vi "gui.vi"(8 "dx":dbl=0.005 format="%#_13g", 9 "f(x)":string[](array[string])=["-sin(x*2*pi(1)) ", "-abs(sin(x*2*pi(1)))", "sin(x*2*pi(1))", "abs(sin(x*2*pi(1)))"], 10 "N":i32=201) -> (2 "y_vals":dbl[][](array[numeric])=[[2.4492935982947064e-16, -0.03141075907812698, -0.06279051952931278, -0.09410831331851353, -0.12533323356430418, -0.15643446504022973, -0.1873813145857242, -0.21814324139654195, -0.24868988716485488, -0.27899110603922833, -0.3090169943749472, -0.338737920245291, -0.3681245526846782, -0.3971478906347799, -0.42577929156507255, -0.4539904997395466, -0.48175367410171566, -0.5090414157503708, -0.5358267949789967, -0.5620833778521305, -0.5877852522924736, -0.6129070536529762, -0.6374239897486899, -0.6613118653236519, -0.6845471059286893, -0.7071067811865474, -0.7289686274214106, -0.7501110696304591, -0.7705132427757893, -0.7901550123756903, -0.8090169943749468, -0.8270805742745616, -0.8443279255020147, -0.8607420270039436, -0.8763066800438631, -0.8910065241883677, -0.9048270524660194, -0.9177546256839813, -0.9297764858882511, -0.9408807689542255, -0.9510565162951535, -0.9602936856769432, -0.968583161128631, -0.9759167619387474, -0.9822872507286886, -0.9876883405951378, -0.9921147013144778, -0.99556196460308, -0.9980267284282716, -0.9995065603657316, -1.0, -0.9995065603657316, -0.9980267284282716, -0.99556196460308, -0.9921147013144779, -0.9876883405951379, -0.9822872507286886, -0.9759167619387473, -0.9685831611286311, -0.9602936856769431, -0.9510565162951536, -0.9408807689542257, -0.9297764858882517, -0.9177546256839815, -0.9048270524660192, -0.8910065241883685, -0.8763066800438634, -0.8607420270039435, -0.8443279255020151, -0.8270805742745619, -0.8090169943749477, -0.7901550123756906, -0.7705132427757897, -0.7501110696304601, -0.728968627421411, -0.7071067811865483, -0.6845471059286897, -0.6613118653236517, -0.6374239897486897, -0.6129070536529766, -0.5877852522924734, -0.562083377852131, -0.5358267949789957, -0.5090414157503721, -0.4817536741017162, -0.4539904997395463, -0.42577929156507394, -0.39714789063478045, -0.368124552684678, -0.33873792024529153, -0.3090169943749478, -0.2789911060392298, -0.2486898871648555, -0.21814324139654168, -0.18738131458572568, -0.15643446504023034, -0.1253332335643039, -0.09410831331851592, -0.06279051952931339, -0.03141075907812848, -3.6739403974420594e-16, 0.03141075907812775, 0.06279051952931265, 0.09410831331851519, 0.12533323356430318, 0.15643446504022962, 0.18738131458572496, 0.2181432413965427, 0.24868988716485477, 0.27899110603922905, 0.30901699437494706, 0.33873792024529253, 0.36812455268467725, 0.3971478906347798, 0.42577929156507327, 0.45399049973954725, 0.48175367410171555, 0.5090414157503714, 0.5358267949789951, 0.5620833778521305, 0.5877852522924728, 0.612907053652976, 0.6374239897486891, 0.6613118653236512, 0.6845471059286892, 0.7071067811865479, 0.7289686274214106, 0.7501110696304596, 0.7705132427757893, 0.7901550123756902, 0.8090169943749472, 0.8270805742745615, 0.8443279255020156, 0.8607420270039432, 0.876306680043863, 0.8910065241883681, 0.9048270524660197, 0.9177546256839811, 0.9297764858882513, 0.9408807689542253, 0.951056516295154, 0.960293685676943, 0.968583161128631, 0.9759167619387472, 0.9822872507286885, 0.9876883405951378, 0.9921147013144779, 0.9955619646030799, 0.9980267284282716, 0.9995065603657316, 1.0, 0.9995065603657316, 0.9980267284282716, 0.9955619646030799, 0.992114701314478, 0.9876883405951379, 0.9822872507286886, 0.9759167619387473, 0.9685831611286312, 0.9602936856769432, 0.9510565162951538, 0.9408807689542251, 0.9297764858882517, 0.9177546256839816, 0.9048270524660192, 0.8910065241883677, 0.8763066800438635, 0.8607420270039436, 0.8443279255020161, 0.8270805742745619, 0.8090169943749477, 0.7901550123756907, 0.7705132427757897, 0.7501110696304601, 0.7289686274214111, 0.7071067811865485, 0.6845471059286898, 0.6613118653236518, 0.6374239897486897, 0.6129070536529767, 0.5877852522924735, 0.5620833778521311, 0.5358267949789958, 0.5090414157503722, 0.4817536741017163, 0.4539904997395464, 0.42577929156507244, 0.39714789063478056, 0.3681245526846781, 0.33873792024529165, 0.3090169943749462, 0.2789911060392299, 0.2486898871648556, 0.21814324139654354, 0.1873813145857258, 0.15643446504023048, 0.125333233564304, 0.09410831331851605, 0.06279051952931351, 0.031410759078128604, 4.898587196589413e-16], [-2.4492935982947064e-16, -0.03141075907812698, -0.06279051952931278, -0.09410831331851353, -0.12533323356430418, -0.15643446504022973, -0.1873813145857242, -0.21814324139654195, -0.24868988716485488, -0.27899110603922833, -0.3090169943749472, -0.338737920245291, -0.3681245526846782, -0.3971478906347799, -0.42577929156507255, -0.4539904997395466, -0.48175367410171566, -0.5090414157503708, -0.5358267949789967, -0.5620833778521305, -0.5877852522924736, -0.6129070536529762, -0.6374239897486899, -0.6613118653236519, -0.6845471059286893, -0.7071067811865474, -0.7289686274214106, -0.7501110696304591, -0.7705132427757893, -0.7901550123756903, -0.8090169943749468, -0.8270805742745616, -0.8443279255020147, -0.8607420270039436, -0.8763066800438631, -0.8910065241883677, -0.9048270524660194, -0.9177546256839813, -0.9297764858882511, -0.9408807689542255, -0.9510565162951535, -0.9602936856769432, -0.968583161128631, -0.9759167619387474, -0.9822872507286886, -0.9876883405951378, -0.9921147013144778, -0.99556196460308, -0.9980267284282716, -0.9995065603657316, -1.0, -0.9995065603657316, -0.9980267284282716, -0.99556196460308, -0.9921147013144779, -0.9876883405951379, -0.9822872507286886, -0.9759167619387473, -0.9685831611286311, -0.9602936856769431, -0.9510565162951536, -0.9408807689542257, -0.9297764858882517, -0.9177546256839815, -0.9048270524660192, -0.8910065241883685, -0.8763066800438634, -0.8607420270039435, -0.8443279255020151, -0.8270805742745619, -0.8090169943749477, -0.7901550123756906, -0.7705132427757897, -0.7501110696304601, -0.728968627421411, -0.7071067811865483, -0.6845471059286897, -0.6613118653236517, -0.6374239897486897, -0.6129070536529766, -0.5877852522924734, -0.562083377852131, -0.5358267949789957, -0.5090414157503721, -0.4817536741017162, -0.4539904997395463, -0.42577929156507394, -0.39714789063478045, -0.368124552684678, -0.33873792024529153, -0.3090169943749478, -0.2789911060392298, -0.2486898871648555, -0.21814324139654168, -0.18738131458572568, -0.15643446504023034, -0.1253332335643039, -0.09410831331851592, -0.06279051952931339, -0.03141075907812848, -3.6739403974420594e-16, -0.03141075907812775, -0.06279051952931265, -0.09410831331851519, -0.12533323356430318, -0.15643446504022962, -0.18738131458572496, -0.2181432413965427, -0.24868988716485477, -0.27899110603922905, -0.30901699437494706, -0.33873792024529253, -0.36812455268467725, -0.3971478906347798, -0.42577929156507327, -0.45399049973954725, -0.48175367410171555, -0.5090414157503714, -0.5358267949789951, -0.5620833778521305, -0.5877852522924728, -0.612907053652976, -0.6374239897486891, -0.6613118653236512, -0.6845471059286892, -0.7071067811865479, -0.7289686274214106, -0.7501110696304596, -0.7705132427757893, -0.7901550123756902, -0.8090169943749472, -0.8270805742745615, -0.8443279255020156, -0.8607420270039432, -0.876306680043863, -0.8910065241883681, -0.9048270524660197, -0.9177546256839811, -0.9297764858882513, -0.9408807689542253, -0.951056516295154, -0.960293685676943, -0.968583161128631, -0.9759167619387472, -0.9822872507286885, -0.9876883405951378, -0.9921147013144779, -0.9955619646030799, -0.9980267284282716, -0.9995065603657316, -1.0, -0.9995065603657316, -0.9980267284282716, -0.9955619646030799, -0.992114701314478, -0.9876883405951379, -0.9822872507286886, -0.9759167619387473, -0.9685831611286312, -0.9602936856769432, -0.9510565162951538, -0.9408807689542251, -0.9297764858882517, -0.9177546256839816, -0.9048270524660192, -0.8910065241883677, -0.8763066800438635, -0.8607420270039436, -0.8443279255020161, -0.8270805742745619, -0.8090169943749477, -0.7901550123756907, -0.7705132427757897, -0.7501110696304601, -0.7289686274214111, -0.7071067811865485, -0.6845471059286898, -0.6613118653236518, -0.6374239897486897, -0.6129070536529767, -0.5877852522924735, -0.5620833778521311, -0.5358267949789958, -0.5090414157503722, -0.4817536741017163, -0.4539904997395464, -0.42577929156507244, -0.39714789063478056, -0.3681245526846781, -0.33873792024529165, -0.3090169943749462, -0.2789911060392299, -0.2486898871648556, -0.21814324139654354, -0.1873813145857258, -0.15643446504023048, -0.125333233564304, -0.09410831331851605, -0.06279051952931351, -0.031410759078128604, -4.898587196589413e-16], [-2.4492935982947064e-16, 0.03141075907812698, 0.06279051952931278, 0.09410831331851353, 0.12533323356430418, 0.15643446504022973, 0.1873813145857242, 0.21814324139654195, 0.24868988716485488, 0.27899110603922833, 0.3090169943749472, 0.338737920245291, 0.3681245526846782, 0.3971478906347799, 0.42577929156507255, 0.4539904997395466, 0.48175367410171566, 0.5090414157503708, 0.5358267949789967, 0.5620833778521305, 0.5877852522924736, 0.6129070536529762, 0.6374239897486899, 0.6613118653236519, 0.6845471059286893, 0.7071067811865474, 0.7289686274214106, 0.7501110696304591, 0.7705132427757893, 0.7901550123756903, 0.8090169943749468, 0.8270805742745616, 0.8443279255020147, 0.8607420270039436, 0.8763066800438631, 0.8910065241883677, 0.9048270524660194, 0.9177546256839813, 0.9297764858882511, 0.9408807689542255, 0.9510565162951535, 0.9602936856769432, 0.968583161128631, 0.9759167619387474, 0.9822872507286886, 0.9876883405951378, 0.9921147013144778, 0.99556196460308, 0.9980267284282716, 0.9995065603657316, 1.0, 0.9995065603657316, 0.9980267284282716, 0.99556196460308, 0.9921147013144779, 0.9876883405951379, 0.9822872507286886, 0.9759167619387473, 0.9685831611286311, 0.9602936856769431, 0.9510565162951536, 0.9408807689542257, 0.9297764858882517, 0.9177546256839815, 0.9048270524660192, 0.8910065241883685, 0.8763066800438634, 0.8607420270039435, 0.8443279255020151, 0.8270805742745619, 0.8090169943749477, 0.7901550123756906, 0.7705132427757897, 0.7501110696304601, 0.728968627421411, 0.7071067811865483, 0.6845471059286897, 0.6613118653236517, 0.6374239897486897, 0.6129070536529766, 0.5877852522924734, 0.562083377852131, 0.5358267949789957, 0.5090414157503721, 0.4817536741017162, 0.4539904997395463, 0.42577929156507394, 0.39714789063478045, 0.368124552684678, 0.33873792024529153, 0.3090169943749478, 0.2789911060392298, 0.2486898871648555, 0.21814324139654168, 0.18738131458572568, 0.15643446504023034, 0.1253332335643039, 0.09410831331851592, 0.06279051952931339, 0.03141075907812848, 3.6739403974420594e-16, -0.03141075907812775, -0.06279051952931265, -0.09410831331851519, -0.12533323356430318, -0.15643446504022962, -0.18738131458572496, -0.2181432413965427, -0.24868988716485477, -0.27899110603922905, -0.30901699437494706, -0.33873792024529253, -0.36812455268467725, -0.3971478906347798, -0.42577929156507327, -0.45399049973954725, -0.48175367410171555, -0.5090414157503714, -0.5358267949789951, -0.5620833778521305, -0.5877852522924728, -0.612907053652976, -0.6374239897486891, -0.6613118653236512, -0.6845471059286892, -0.7071067811865479, -0.7289686274214106, -0.7501110696304596, -0.7705132427757893, -0.7901550123756902, -0.8090169943749472, -0.8270805742745615, -0.8443279255020156, -0.8607420270039432, -0.876306680043863, -0.8910065241883681, -0.9048270524660197, -0.9177546256839811, -0.9297764858882513, -0.9408807689542253, -0.951056516295154, -0.960293685676943, -0.968583161128631, -0.9759167619387472, -0.9822872507286885, -0.9876883405951378, -0.9921147013144779, -0.9955619646030799, -0.9980267284282716, -0.9995065603657316, -1.0, -0.9995065603657316, -0.9980267284282716, -0.9955619646030799, -0.992114701314478, -0.9876883405951379, -0.9822872507286886, -0.9759167619387473, -0.9685831611286312, -0.9602936856769432, -0.9510565162951538, -0.9408807689542251, -0.9297764858882517, -0.9177546256839816, -0.9048270524660192, -0.8910065241883677, -0.8763066800438635, -0.8607420270039436, -0.8443279255020161, -0.8270805742745619, -0.8090169943749477, -0.7901550123756907, -0.7705132427757897, -0.7501110696304601, -0.7289686274214111, -0.7071067811865485, -0.6845471059286898, -0.6613118653236518, -0.6374239897486897, -0.6129070536529767, -0.5877852522924735, -0.5620833778521311, -0.5358267949789958, -0.5090414157503722, -0.4817536741017163, -0.4539904997395464, -0.42577929156507244, -0.39714789063478056, -0.3681245526846781, -0.33873792024529165, -0.3090169943749462, -0.2789911060392299, -0.2486898871648556, -0.21814324139654354, -0.1873813145857258, -0.15643446504023048, -0.125333233564304, -0.09410831331851605, -0.06279051952931351, -0.031410759078128604, -4.898587196589413e-16], [2.4492935982947064e-16, 0.03141075907812698, 0.06279051952931278, 0.09410831331851353, 0.12533323356430418, 0.15643446504022973, 0.1873813145857242, 0.21814324139654195, 0.24868988716485488, 0.27899110603922833, 0.3090169943749472, 0.338737920245291, 0.3681245526846782, 0.3971478906347799, 0.42577929156507255, 0.4539904997395466, 0.48175367410171566, 0.5090414157503708, 0.5358267949789967, 0.5620833778521305, 0.5877852522924736, 0.6129070536529762, 0.6374239897486899, 0.6613118653236519, 0.6845471059286893, 0.7071067811865474, 0.7289686274214106, 0.7501110696304591, 0.7705132427757893, 0.7901550123756903, 0.8090169943749468, 0.8270805742745616, 0.8443279255020147, 0.8607420270039436, 0.8763066800438631, 0.8910065241883677, 0.9048270524660194, 0.9177546256839813, 0.9297764858882511, 0.9408807689542255, 0.9510565162951535, 0.9602936856769432, 0.968583161128631, 0.9759167619387474, 0.9822872507286886, 0.9876883405951378, 0.9921147013144778, 0.99556196460308, 0.9980267284282716, 0.9995065603657316, 1.0, 0.9995065603657316, 0.9980267284282716, 0.99556196460308, 0.9921147013144779, 0.9876883405951379, 0.9822872507286886, 0.9759167619387473, 0.9685831611286311, 0.9602936856769431, 0.9510565162951536, 0.9408807689542257, 0.9297764858882517, 0.9177546256839815, 0.9048270524660192, 0.8910065241883685, 0.8763066800438634, 0.8607420270039435, 0.8443279255020151, 0.8270805742745619, 0.8090169943749477, 0.7901550123756906, 0.7705132427757897, 0.7501110696304601, 0.728968627421411, 0.7071067811865483, 0.6845471059286897, 0.6613118653236517, 0.6374239897486897, 0.6129070536529766, 0.5877852522924734, 0.562083377852131, 0.5358267949789957, 0.5090414157503721, 0.4817536741017162, 0.4539904997395463, 0.42577929156507394, 0.39714789063478045, 0.368124552684678, 0.33873792024529153, 0.3090169943749478, 0.2789911060392298, 0.2486898871648555, 0.21814324139654168, 0.18738131458572568, 0.15643446504023034, 0.1253332335643039, 0.09410831331851592, 0.06279051952931339, 0.03141075907812848, 3.6739403974420594e-16, 0.03141075907812775, 0.06279051952931265, 0.09410831331851519, 0.12533323356430318, 0.15643446504022962, 0.18738131458572496, 0.2181432413965427, 0.24868988716485477, 0.27899110603922905, 0.30901699437494706, 0.33873792024529253, 0.36812455268467725, 0.3971478906347798, 0.42577929156507327, 0.45399049973954725, 0.48175367410171555, 0.5090414157503714, 0.5358267949789951, 0.5620833778521305, 0.5877852522924728, 0.612907053652976, 0.6374239897486891, 0.6613118653236512, 0.6845471059286892, 0.7071067811865479, 0.7289686274214106, 0.7501110696304596, 0.7705132427757893, 0.7901550123756902, 0.8090169943749472, 0.8270805742745615, 0.8443279255020156, 0.8607420270039432, 0.876306680043863, 0.8910065241883681, 0.9048270524660197, 0.9177546256839811, 0.9297764858882513, 0.9408807689542253, 0.951056516295154, 0.960293685676943, 0.968583161128631, 0.9759167619387472, 0.9822872507286885, 0.9876883405951378, 0.9921147013144779, 0.9955619646030799, 0.9980267284282716, 0.9995065603657316, 1.0, 0.9995065603657316, 0.9980267284282716, 0.9955619646030799, 0.992114701314478, 0.9876883405951379, 0.9822872507286886, 0.9759167619387473, 0.9685831611286312, 0.9602936856769432, 0.9510565162951538, 0.9408807689542251, 0.9297764858882517, 0.9177546256839816, 0.9048270524660192, 0.8910065241883677, 0.8763066800438635, 0.8607420270039436, 0.8443279255020161, 0.8270805742745619, 0.8090169943749477, 0.7901550123756907, 0.7705132427757897, 0.7501110696304601, 0.7289686274214111, 0.7071067811865485, 0.6845471059286898, 0.6613118653236518, 0.6374239897486897, 0.6129070536529767, 0.5877852522924735, 0.5620833778521311, 0.5358267949789958, 0.5090414157503722, 0.4817536741017163, 0.4539904997395464, 0.42577929156507244, 0.39714789063478056, 0.3681245526846781, 0.33873792024529165, 0.3090169943749462, 0.2789911060392299, 0.2486898871648556, 0.21814324139654354, 0.1873813145857258, 0.15643446504023048, 0.125333233564304, 0.09410831331851605, 0.06279051952931351, 0.031410759078128604, 4.898587196589413e-16]], 3 "cancelled":bool=TRUE)   [LabVIEW 2017, in "wf.lvlib"]
uses:
  wf.lvlib
  wf_output.ctl
  <vilib>/Utility/xml.llb/Write to XML File(string).vi
  <vilib>/Utility/xml.llb/Read From XML File(string).vi
  tools/tools.lvlib
panel:
  in  "Tab Control":enum32{"plot", "funcs", "output", "devices"}(tab)
  out "Waveform Graph":waveform(dbl)[](graph)=[{"t0"=timestamp(0 s since 1904-01-01), "dt"=0.005, "Y"=array[201 elements]}, {"t0"=timestamp(0 s since 1904-01-01), "dt"=0.005, "Y"=array[201 elements]}, {"t0"=timestamp(0 s since 1904-01-01), "dt"=0.005, "Y"=array[201 elements]}, {"t0"=timestamp(0 s since 1904-01-01), "dt"=0.005, "Y"=array[201 elements]}]
  in  "output":T1[](array[typedef])=[{"rate (Sa / s)"=20000000.0, "amp (V)"=0.1, "offset (V)"=0.0}, {"rate (Sa / s)"=20000000.0, "amp (V)"=0.05, "offset (V)"=0.0}]
  in  "wf_multi":T2(array[cluster])=[{"device"="waveform_gen", "chan"=1}, {"device"="waveform_gen", "chan"=2}] {"chan" items=["1"=1, "2"=2]}
  in  "upload":bool
  in  "quit":bool
  in  "load":bool
  in  "save":bool
  in  "build":bool
  # "(arb.)"
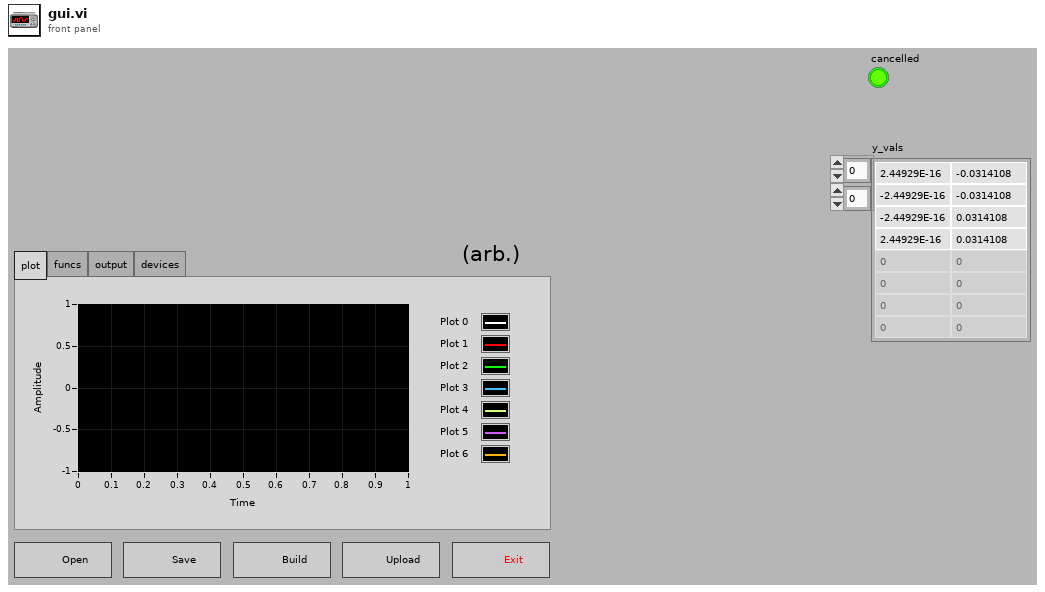
[diagram p1: front panel]
types:
  T1 = typedef "wf.lvlib/wf_output.ctl" = cluster{"rate (Sa / s)":dbl, "amp (V)":dbl, "offset (V)":dbl}
  T2 = cluster{"device":refnum<visa-resource-name>, "chan":i32}[]
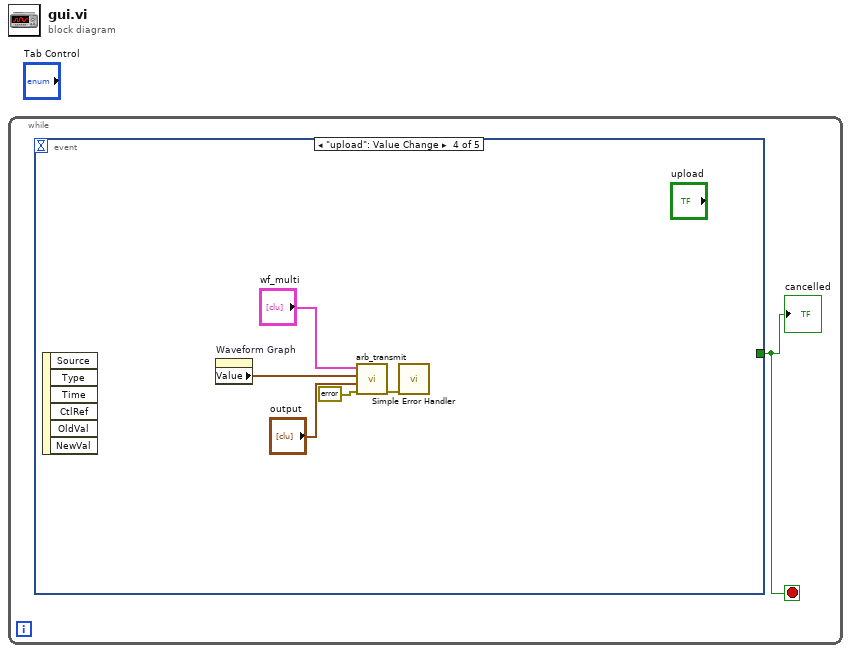
[diagram p0: block diagram]
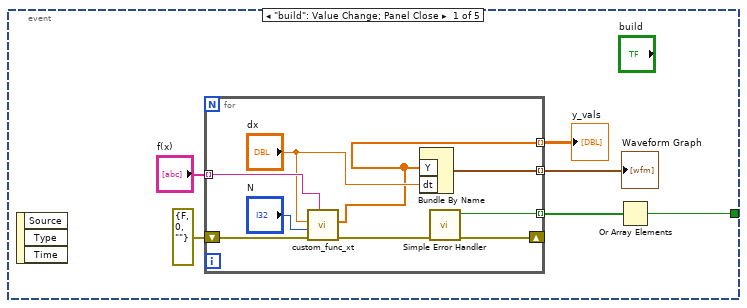
[diagram p2: hidden frame]
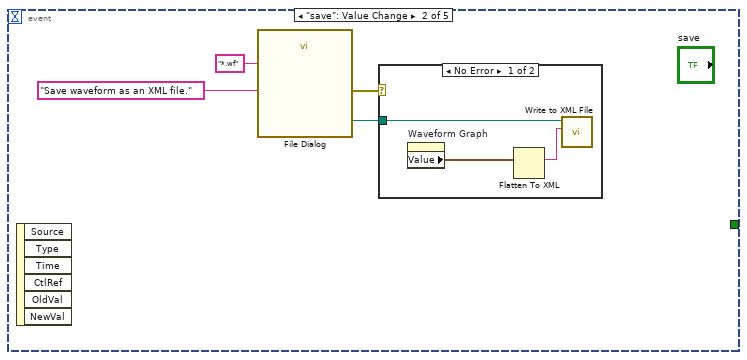
[diagram p3: hidden frame]
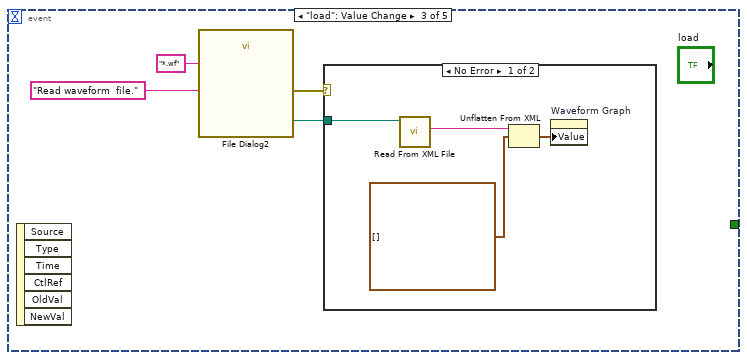
[diagram p5: hidden frame]
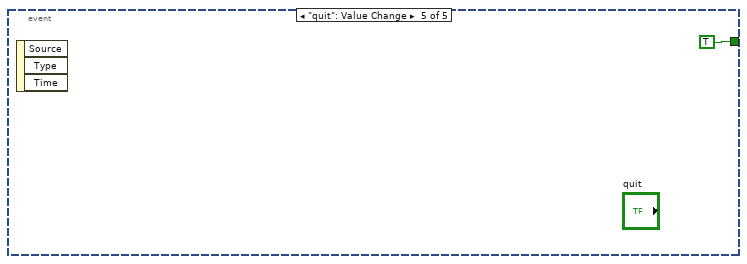
[diagram p7: hidden frame]
diagram:
  n1 = while {
    stop <- w1 stop-if-true
    n2 = event shown="[3] \"upload\": Value Change" {
      selector: _ -> [_ _ _ _ _]
      dyn-events: _ -> [_ _ _ _ _]
      timeout: _ -> [_ _ _ _ _]
      tunnel: [w4 _ _ _ TRUE ("Cancel")] -> w1
      event "build": Value Change; Panel Close {
        n3 = event-data() -> ()  [unwired: 1 in, 3 out]
        n4 = for {
          tunnel: [w14] -> w5 mode=indexing
          shift-right: [w13] -> _
          shift-left: errorcluster {"status"=FALSE, "code"=0, "source"=""} ("error in (no error)") -> [w12]
          tunnel: "f(x)" -> [w11] mode=indexing
          tunnel: [w8] -> w3 mode=indexing
          tunnel: [w9] -> w2 mode=indexing
          n5 = call "custom_func_xt.vi"("func"=w11, "error in (no error)"=w12, "N"="N", "dx"="dx") -> ("error out"=w15:errorcluster, "y_vals"=w8:dbl[])  [unwired: 6 in]
          n6 = Bundle By Name("Y"=w8, "dt"="dx") -> (w9:waveform(dbl))  [unwired: 1 in]
          n7 = call <vilib>:"Simple Error Handler.vi"("error in (no error)"=w15) -> ("error?"=w14:bool, "error out"=w13:errorcluster)  [unwired: 4 in, 3 out]
        }
        "y_vals" <- w3
        "Waveform Graph" <- w2
        n8 = Or Array Elements(Boolean array=w5) -> (logical OR=w4:bool)
      }
      event "save": Value Change {
        n9 = event-data() -> ()  [unwired: 1 in, 6 out]
        n10 = call "File Dialog"("prompt"="Save waveform as an XML file.", "pattern (all files)"="*.wf" ("pattern label")) -> ("selected path"=w20:path, "error out"=w17:errorcluster)  [unwired: 10 in, 2 out]
        n11 = case shown="No Error" w17 {
          tunnel: w20 -> [w22 _]
          frame No Error {
            n12 = property on="Waveform Graph" class="WFGraph (strict)"() -> ("Value"=w21:waveform(dbl)[])  [unwired: 2 in, 2 out]
            n13 = Flatten To XML(anything=w21) -> (xml string=w23:string)
            n14 = call-poly <vilib>:"Write to XML File.vi"("XML Input"=w23, "XML File Path"=w22) -> ()  [unwired: 7 in, 3 out]
          }
          frame Error {
          }
        }
      }
      event "load": Value Change {
        n15 = event-data() -> ()  [unwired: 1 in, 6 out]
        n16 = call "File Dialog2"("prompt"="Read waveform  file.", "pattern (all files)"="*.wf" ("pattern label")) -> ("selected path"=w25:path, "error out"=w24:errorcluster)  [unwired: 10 in, 2 out]
        n17 = case shown="No Error" w24 {
          tunnel: w25 -> [w31 _]
          frame No Error {
            n18 = call-poly <vilib>:"Read From XML File.vi"("XML File Path"=w31) -> ("XML Elements"=w30:string)  [unwired: 8 in, 2 out]
            n19 = Unflatten From XML(xml string=w30, type=waveform(dbl)[] [] ("electrodes 2")) -> (value=w28:waveform(dbl)[])  [unwired: 1 in, 1 out]
            n20 = property on="Waveform Graph" class="WFGraph (strict)"("Value"=w28) -> ()  [unwired: 2 in, 2 out]
          }
          frame Error {
          }
        }
      }
      event "upload": Value Change {
        n21 = event-data() -> ()  [unwired: 1 in, 6 out]
        n22 = property on="Waveform Graph" class="WFGraph (strict)"() -> ("Value"=w36:waveform(dbl)[])  [unwired: 2 in, 2 out]
        n23 = call "arb_transmit.vi"("error in (no error)"=errorcluster {"status"=FALSE, "code"=0, "source"=""}, "output"="output", "Waveform Graph"=w36, "VISA"="wf_multi") -> ("error out"=w35:errorcluster)  [unwired: 7 in]
        n24 = call <vilib>:"Simple Error Handler.vi"("error in (no error)"=w35) -> ()  [unwired: 4 in, 5 out]
      }
      event "quit": Value Change {
        n25 = event-data() -> ()  [unwired: 1 in, 3 out]
      }
    }
    "cancelled" <- w1
  }
